vi "Simple add.vi"() -> ()   [LabVIEW 2016]
panel:
  in  "Z":dbl
  out "x+y+z":dbl
  in  "x":dbl
  in  "y":dbl
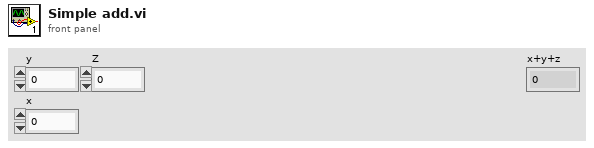
[diagram p1: front panel]
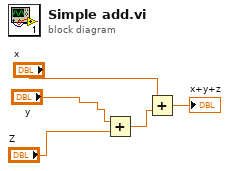
[diagram p0: block diagram]
diagram:
  n1 = Add(x="y", y="Z") -> (x+y=w1:dbl)
  n2 = Add(x="x", y=w1) -> (x+y=→"x+y+z":dbl)
